vi "TDC_DAQV33_Paralled_muon.vi"(7 "address":string[](array[string])=["192.168.10.29"], 8 "error in (no error)":errorcluster, 9 "stop":bool, 10 "save data":bool=TRUE, 11 "SMA mode":bool) -> (0 "error out 3":errorcluster, 2 "csv path":path=path "G:/tdc/2017/data/test_20250707_095708.csv", 3 "rate":dbl=0.9919403977777173)   [LabVIEW 2017]
uses:
  gloabal.vi
  <vilib>/Utility/file.llb/Write Delimited Spreadsheet (DBL).vi
  <vilib>/Utility/file.llb/Write Delimited Spreadsheet (I64).vi
panel:
  in  "append csv 2":bool
  out "pmt trigger rate":u32[](array[numeric])=[0, 0, 1000, 0, 0, 0, 0, 0, 0, 0, 0, 0, 0, 0, 0, 0, 0, 0, 0, 0, 0, 0, 0, 0, 0, 0, 0, 0, 0, 0, 0, 0, 0, 0, 0, 0, 0, 0, 0, 0, 0, 0, 0, 0, 0, 0, 0, 0, 0, 0, 0, 0, 0, 0, 0, 0, 0, 0, 0, 0, 0, 0, 0, 0]
  out "event":u32[](array[numeric])=[0, 0, 0, 0, 1060, 1060, 0, 0, 0, 0, 0, 0, 0, 0, 0, 0, 0, 0, 0, 0, 0, 0, 0, 0, 0, 0, 0, 0, 0, 0, 0, 0, 0, 0, 0, 0, 0, 0, 0, 0, 0, 0, 0, 0, 0, 0, 0, 0, 0, 0, 0, 0, 0, 0, 0, 0, 0, 0, 0, 0, 0, 0, 0, 0, 0, 0, 0, 0, 0, 0, 0, 0, 0, 0, 0, 0, 0, 0, 0, 0, 0, 0, 0, 0, 0, 0, 0, 0, 0, 0, 0, 0, 0, 0, 0, 0, 0, 0, 0, 0, 0, 0, 0, 0, 0, 0, 0, 0, 0, 0, 0, 0, 0, 0, 0, 0, 0, 0, 0, 0, 0, 0, 0, 0, 0, 0, 0, 0]
  in  "calib_file":path=path "G:/tdc/2017/data/112_20250410_codeDensity.csv" caption="文件路径 （空时为对话框）"
  in  "use_calib_file":bool=TRUE
  out "second stamp":u64
  in  "coarse counter width":u16(ring) items=["29", "48"]
  out "name (unnamed)":string="Z\t"
  out "error out 5":errorcluster
  in  "timeout":dbl=30000.0
  out "DAC":dbl=8094.0
  out "Out":u8=3 format="%.0x"
  out "coarse":u64=407532724 format="%x"
  in  "gps":bool
  out "Year":string="2025"
  in  "factor":i32=128
  in  "displayCR":bool=TRUE
  in  "Counter Setting":dbl=100000.0 format="%#_13g"
  in  "replace dat":bool
  in  "append csv":bool=TRUE
  out "element":string
  out "fine":u64=646 format="%x"
  in  "UDP Config":bool=TRUE
  in  "data  path":path=path "G:/tdc/2017/data"
  out "cal 2":u64[](graph)
  in  "Thresholds (mV)":dbl[](array[numeric])=[580.0, 580.0, 580.0, 580.0, 600.0, 600.0, 600.0, 600.0, 580.0, 580.0, 600.0, 600.0, 600.0, 600.0, 600.0, 600.0, 580.0, 580.0, 600.0, 600.0, 600.0, 600.0, 600.0, 600.0, 580.0, 580.0, 600.0, 600.0, 600.0, 600.0, 600.0, 600.0, 600.0, 600.0, 600.0, 600.0, 600.0, 600.0, 600.0, 600.0, 600.0, 600.0, 600.0, 600.0, 600.0, 600.0, 600.0, 600.0, 600.0, 600.0, 600.0, 600.0, 600.0, 600.0, 600.0, 600.0, 600.0, 600.0, 600.0, 600.0, 600.0, 600.0, 600.0, 600.0]
  out "error out 2":errorcluster
  in  "display":bool=TRUE
  in  "Thresholds":dbl=-0.03
  in  "one key for threshold":bool=TRUE
  in  "RST":bool
  in  "通道数量":i32=128
  out "Cal Table":u32[](array[numeric])=[100002, 100002, 100002, 100002, 100002, 100002, 100002, 100002, 100002, 100002, 100002, 100002, 100002, 100002, 100002, 100002, 100002, 100002, 100002, 100002, 100002, 100002, 100002, 100002, 100002, 100002, 100002, 100002, 100002, 100002, 100002, 100002, 100002, 100002, 100002, 100002, 100002, 100002, 100002, 100002, 100002, 100002, 100002, 100002, 100002, 100002, 100002, 100002, 100002, 100002, 100002, 100002, 100002, 100002, 100002, 100002, 100002, 100002, 100002, 100002, 100002, 100002, 100002, 100002, 100002, 100002, 100002, 100002, 100002, 100002, 100002, 100002, 100002, 100002, 100002, 100002, 100002, 100002, 100002, 100002, 100002, 100002, 100002, 100002, 100002, 100002, 100002, 100002, 100002, 100002, 100002, 100002, 100002, 100002, 100002, 100002, 100002, 100002, 100002, 100002, 100002, 100002, 100002, 100002, 100002, 100002, 100002, 100002, 100002, 100002, 100002, 100002, 100002, 100002, 100002, 100002, 100002, 100002, 100002, 100002, 100002, 100002, 100002, 100002, 100002, 100002, 100002, 100002]
  in  "channel for cal":i32
  out "channel number":u64=5
  out "Calibration Counter":i32=536
  out "Event index":i32=97959
  out "cal":i64[](graph)=[0, 0, 0, 0, 0, 0, 0, 0, 0, 0, 0, 0, 0, 0, 0, 0, 0, 0, 0, 0, 0, 0, 0, 0, 0, 0, 0, 0, 0, 0, 0, 0, 0, 0, 0, 0, 0, 0, 0, 0, 0, 0, 0, 0, 0, 0, 0, 0, 0, 0, 0, 0, 0, 0, 0, 0, 0, 0, 0, 0, 0, 0, 0, 0, 0, 0, 0, 0, 0, 0, 0, 0, 0, 0, 0, 0, 0, 0, 0, 0, 0, 0, 0, 0, 0, 0, 0, 0, 0, 0, 0, 0, 0, 0, 0, 0, 0, 0, 0, 0, 0, 0, 0, 0, 0, 0, 0, 0, 0, 0, 0, 0, 0, 0, 0, 0, 0, 0, 0, 0, 0, 0, 0, 0, 0, 0, 0, 0, 0, 0, 0, 0, 0, 0, 0, 0, 0, 1, 76, 599, 343, 108, 71, 417, 154, 260, 138, 496, 255, 81, 42, 120, 215, 68, 109, 755, 65, 198, 68, 46, 289, 113, 477, 47, 391, 38, 57, 219, 61, 197, 92, 551, 105, 63, 72, 376, 118, 80, 104, 342, 66, 364, 53, 205, 180, 55, 61, 98, 566, 70, 259, 156, 66, 67, 62, 104, 344, 46, 318, 61, 43, 100, 186, 168, 212, 388, 97, 172, 75, 128, 55, 98, 77, 117, 184, 418, 122, 97, 132, 56, 45, 166, 426, 71, 70, 199, 69, 200, 161, 248, 119, 436, 79, 44, 50, 173, 567, 316, 65, 121, 253, 131, 217, 41, 55, 98, 38, 288, 113, 48, 254, 53, 28, 49, 132, 59, 311, 49, 49, 130, 54, 36, 46, 50, 158, 319, 298, 204, 87, 114, 100, 329, 92, 156, 15, 137, 321, 63, 192, 111, 45, 54, 43, 44, 598, 220, 210, 106, 235, 55, 49, 53, 377, 47, 32, 49, 50, 351, 179, 270, 239, 267, 89, 121, 85, 226, 33, 24, 25, 72, 480, 43, 48, 235, 221, 48, 66, 40, 422, 151, 110, 151, 177, 231, 74, 69, 108, 173, 239, 91, 371, 76, 80, 66, 459, 75, 238, 263, 522, 79, 63, 34, 80, 39, 64, 330, 323, 495, 47, 37, 33, 47, 399, 35, 32, 31, 100, 83, 44, 232, 44, 93, 144, 317, 125, 80, 64, 134, 85, 45, 156, 214, 71, 67, 406, 77, 45, 28, 35, 55, 136, 169, 99, 256, 128, 536, 80, 81, 92, 242, 165, 190, 64, 42, 72, 107, 301, 43, 55, 156, 281, 71, 245, 161, 73, 57, 387, 108, 146, 208, 61, 102, 266, 55, 224, 185, 56, 40, 83, 584, 66, 58, 46, 117, 163, 61, 303, 75, 85, 192, 150, 166, 72, 64, 161, 355, 147, 59, 195, 86, 71, 191, 55, 66, 353, 300, 73, 93, 202, 120, 66, 112, 284, 377, 166, 78, 145, 137, 190, 61, 48, 54, 277, 221, 458, 61, 69, 47, 366, 116, 215, 163, 64, 211, 129, 143, 119, 203, 426, 147, 228, 124, 116, 34, 101, 218, 59, 150, 117, 180, 58, 87, 231, 77, 150, 58, 106, 60, 226, 46, 46, 52, 371, 114, 275, 43, 41, 119, 67, 150, 60, 323, 211, 56, 94, 364, 108, 215, 52, 49, 150, 249, 240, 74, 119, 56, 298, 214, 132, 68, 81, 250, 114, 348, 87, 138, 63, 80, 423, 63, 67, 85, 224, 73, 245, 83, 38, 37, 181, 65, 312, 437, 138, 117, 42, 43, 105, 253, 82, 63, 86, 51, 175, 390, 48, 55, 377, 69, 117, 86, 498, 60, 54, 166, 214, 53, 100, 165, 77, 101, 205, 249, 342, 96, 522, 78, 45, 289, 230, 164, 363, 47, 56, 133, 76, 99, 133, 364, 83, 297, 109, 118, 78, 46, 35, 53, 215, 107, 62, 92, 81, 368, 47, 60, 168, 57, 110, 71, 58, 559, 141, 67, 113, 284, 287, 261, 134, 73, 53, 318, 104, 156, 632, 39, 27, 42, 433, 326, 279, 111, 229, 73, 91, 258, 88, 180, 213, 107, 329, 211, 54, 202, 126, 60, 149, 116, 154, 90, 68, 53, 73, 53, 199, 223, 118, 68, 152, 90, 197, 104, 49, 83, 340, 263, 86, 80, 100, 225, 475, 104, 160, 119, 248, 157, 81, 204, 157, 139, 99, 266, 82, 38, 71, 203, 458, 99, 186, 77, 115, 67, 353, 58, 37, 409, 84, 60, 85, 83, 96, 212, 161, 411, 374, 66, 44, 66, 84, 120, 196, 33, 35, 61, 205, 418, 169, 58, 95, 84, 34, 220, 84, 92, 239, 105, 273, 220, 55, 414, 81, 129, 130, 96, 165, 75, 393, 336, 170, 64, 84, 76, 386, 679, 76, 57, 161, 55, 76, 374, 268, 134, 206, 91, 61, 55, 395, 367, 166, 65, 35, 56, 224, 59, 92, 116, 197, 126, 121, 126, 63, 85, 138, 56, 11, 109, 5, 0, 1, 0, 0, 0, 0, 0, 0, 0, 0, 0, 0, 0, 0, 0, 0, 0, 0, 0, 0, 0, 0, 0, 0, 0, 0, 0, 0, 0, 0, 0, 0, 0, 0, 0, 0, 0, 0, 0, 0, 0, 0, 0, 0, 0, 0, 0, 0, 0, 0, 0, 0, 0, 0, 0, 0, 0, 0, 0, 0, 0, 0, 0, 0, 0, 0, 0, 0, 0, 0, 0, 0, 0, 0, 0, 0, 0, 0, 0, 0, 0, 0, 0, 0, 0, 0, 0, 0, 0, 0, 0, 0, 0, 0, 0, 0, 0, 0, 0, 0, 0, 0, 0, 0, 0, 0, 0, 0, 0, 0, 0, 0, 0, 0, 0, 0, 0, 0, 0, 0, 0, 0, 0, 0, 0, 0, 0, 0, 0, 0, 0, 0, 0, 0, 0, 0, 0, 0, 0, 0, 0, 0, 0, 0, 0, 0, 0, 0, 0, 0, 0, 0, 0, 0, 0, 0, 0, 0, 0, 0, 0, 0, 0, 0, 0, 0, 0, 0, 0, 0, 0, 0, 0, 0, 0, 0, 0, 0, 0, 0, 0, 0, 0, 0, 0, 0, 0, 0, 0, 0, 0, 0, 0, 0, 0, 0, 0, 0, 0, 0, 0, 0, 0, 0, 0, 0, 0, 0, 0, 0, 0, 0, 0, 0, 0, 0, 0, 0, 0, 0, 0, 0, 0, 0, 0, 0, 0, 0, 0, 0, 0, 0, 0, 0, 0, 0, 0, 0, 0, 0, 0, 0, 0, 0, 0, 0, 0, 0, 0, 0, 0, 0, 0, 0, 0, 0, 0, 0, 0, 0, 0, 0, 0, 0, 0, 0, 0, 0, 0, 0, 0, 0, 0, 0, 0, 0, 0, 0, 0, 0, 0, 0, 0, 0, 0, 0, 0, 0, 0, 0, 0, 0, 0, 0, 0, 0, 0, 0, 0, 0, 0, 0, 0, 0, 0, 0, 0, 0, 0, 0, 0, 0, 0, 0, 0, 0, 0, 0, 0, 0, 0, 0, 0, 0, 0, 0, 0, 0, 0, 0, 0, 0, 0, 0, 0, 0, 0, 0, 0, 0, 0, 0, 0, 0, 0, 0, 0, 0, 0, 0, 0, 0, 0, 0, 0, 0, 0, 0, 0, 0, 0, 0, 0, 0, 0, 0, 0, 0, 0, 0, 0, 0, 0, 0, 0, 0, 0, 0, 0, 0, 0, 0, 0, 0, 0, 0, 0, 0, 0, 0, 0, 0, 0, 0, 0, 0, 0, 0, 0, 0, 0, 0, 0, 0, 0, 0, 0, 0, 0, 0, 0, 0, 0, 0, 0, 0, 0, 0, 0, 0, 0, 0, 0, 0, 0, 0, 0, 0, 0, 0, 0, 0, 0, 0, 0, 0, 0, 0, 0, 0, 0, 0, 0, 0, 0, 0, 0, 0, 0, 0, 0, 0, 0, 0, 0, 0, 0, 0, 0, 0, 0, 0, 0, 0, 0, 0, 0, 0, 0, 0, 0, 0, 0, 0, 0, 0, 0, 0, 0, 0, 0, 0, 0, 0, 0, 0, 0, 0, 0, 0, 0, 0, 0, 0, 0, 0, 0, 0, 0, 0, 0, 0, 0, 0, 0, 0, 0, 0, 0, 0, 0, 0, 0, 0, 0, 0, 0, 0, 0, 0, 0, 0, 0, 0, 0, 0, 0, 0, 0, 0, 0, 0, 0, 0, 0, 0, 0, 0, 0, 0, 0, 0, 0, 0, 0, 0, 0, 0, 0, 0, 0, 0, 0, 0, 0, 0, 0, 0, 0, 0, 0, 0, 0, 0, 0, 0, 0, 0, 0, 0, 0, 0, 0, 0, 0, 0, 0, 0, 0, 0, 0, 0, 0, 0, 0, 0, 0, 0, 0, 0, 0, 0, 0, 0, 0, 0, 0, 0, 0, 0, 0, 0, 0, 0, 0, 0, 0, 0, 0, 0, 0, 0, 0, 0, 0, 0, 0, 0, 0, 0, 0, 0, 0, 0, 0, 0, 0, 0, 0, 0, 0, 0, 0, 0, 0, 0, 0, 0, 0, 0, 0, 0, 0, 0, 0, 0, 0, 0, 0, 0, 0, 0, 0, 0, 0, 0, 0, 0, 0, 0, 0, 0, 0, 0, 0, 0, 0, 0, 0, 0, 0, 0, 0, 0, 0, 0, 0, 0, 0, 0, 0, 0, 0, 0, 0, 0, 0, 0, 0, 0, 0, 0, 0, 0, 0, 0, 0, 0, 0, 0, 0, 0, 0, 0, 0, 0, 0, 0, 0, 0, 0, 0, 0, 0, 0, 0, 0, 0, 0, 0, 0, 0, 0, 0, 0, 0, 0, 0, 0, 0, 0, 0, 0, 0, 0, 0, 0, 0, 0, 0, 0, 0, 0, 0, 0, 0, 0, 0, 0, 0, 0, 0, 0, 0, 0, 0, 0, 0, 0, 0, 0, 0, 0, 0, 0, 0, 0, 0, 0, 0, 0, 0, 0, 0, 0, 0, 0, 0, 0, 0, 0, 0, 0, 0, 0, 0, 0, 0, 0, 0, 0, 0, 0, 0, 0, 0, 0, 0, 0, 0, 0, 0, 0, 0, 0, 0, 0, 0, 0, 0, 0, 0, 0, 0, 0, 0, 0, 0, 0, 0, 0, 0, 0, 0, 0, 0, 0, 0, 0, 0, 0, 0, 0, 0, 0, 0, 0, 0, 0, 0, 0, 0, 0, 0, 0, 0, 0, 0, 0, 0, 0, 0, 0, 0, 0, 0, 0, 0, 0, 0, 0, 0, 0, 0, 0, 0, 0, 0, 0, 0, 0, 0, 0, 0, 0, 0, 0, 0, 0, 0, 0, 0, 0, 0, 0, 0, 0, 0, 0, 0, 0, 0, 0, 0, 0, 0, 0, 0, 0, 0, 0, 0, 0, 0, 0, 0, 0, 0, 0, 0, 0, 0, 0, 0, 0, 0, 0, 0, 0, 0, 0, 0, 0, 0, 0, 0, 0, 0, 0, 0, 0, 0, 0, 0, 0, 0, 0, 0, 0, 0, 0, 0, 0, 0, 0, 0, 0, 0, 0, 0, 0, 0, 0, 0, 0, 0, 0, 0, 0, 0, 0, 0, 0, 0, 0, 0, 0, 0, 0, 0, 0, 0, 0, 0, 0, 0, 0, 0, 0, 0, 0, 0, 0, 0, 0, 0, 0, 0, 0, 0, 0, 0, 0, 0, 0, 0, 0, 0, 0, 0, 0, 0, 0, 0, 0, 0, 0, 0, 0, 0, 0, 0, 0, 0, 0, 0, 0, 0, 0, 0, 0, 0, 0, 0, 0, 0, 0, 0, 0, 0, 0, 0, 0, 0, 0, 0, 0, 0, 0, 0, 0, 0, 0, 0, 0, 0, 0, 0, 0, 0, 0, 0, 0, 0, 0, 0, 0, 0, 0, 0, 0, 0, 0, 0, 0, 0, 0, 0, 0, 0, 0, 0, 0, 0, 0, 0, 0, 0, 0, 0, 0, 0, 0, 0, 0, 0, 0, 0, 0, 0, 0, 0, 0, 0, 0, 0, 0, 0, 0, 0, 0, 0, 0, 0, 0, 0, 0, 0, 0, 0, 0, 0, 0, 0, 0, 0, 0, 0, 0, 0, 0, 0, 0, 0, 0, 0, 0, 0, 0, 0, 0, 0, 0, 0, 0, 0, 0, 0, 0, 0, 0, 0, 0, 0, 0, 0, 0, 0, 0, 0, 0, 0, 0, 0, 0, 0, 0, 0, 0, 0, 0, 0, 0, 0, 0, 0, 0, 0, 0, 0, 0, 0, 0, 0, 0, 0, 0, 0, 0, 0, 0, 0, 0, 0, 0, 0, 0, 0, 0, 0, 0, 0, 0, 0, 0, 0, 0, 0, 0, 0, 0, 0, 0, 0, 0, 0, 0, 0, 0, 0, 0, 0, 0, 0, 0, 0, 0, 0, 0, 0, 0, 0, 0, 0, 0, 0, 0, 0, 0, 0, 0, 0, 0, 0, 0, 0, 0, 0, 0, 0, 0, 0, 0, 0, 0, 0, 0, 0, 0, 0, 0, 0, 0, 0, 0, 0, 0, 0, 0, 0, 0, 0, 0]
  out "error out":errorcluster={"status"=TRUE, "code"=1, "source"="Close File in TDC_DAQV33_Paralled_muon.vi"}
  out "appended path":path=path "G:/tdc/2017/data/test_20250707_095708.dat"
  in  "filename":string="test"
  in  "Events":i32=110000 min=1
  in  "timeout (ms)":i32=10000
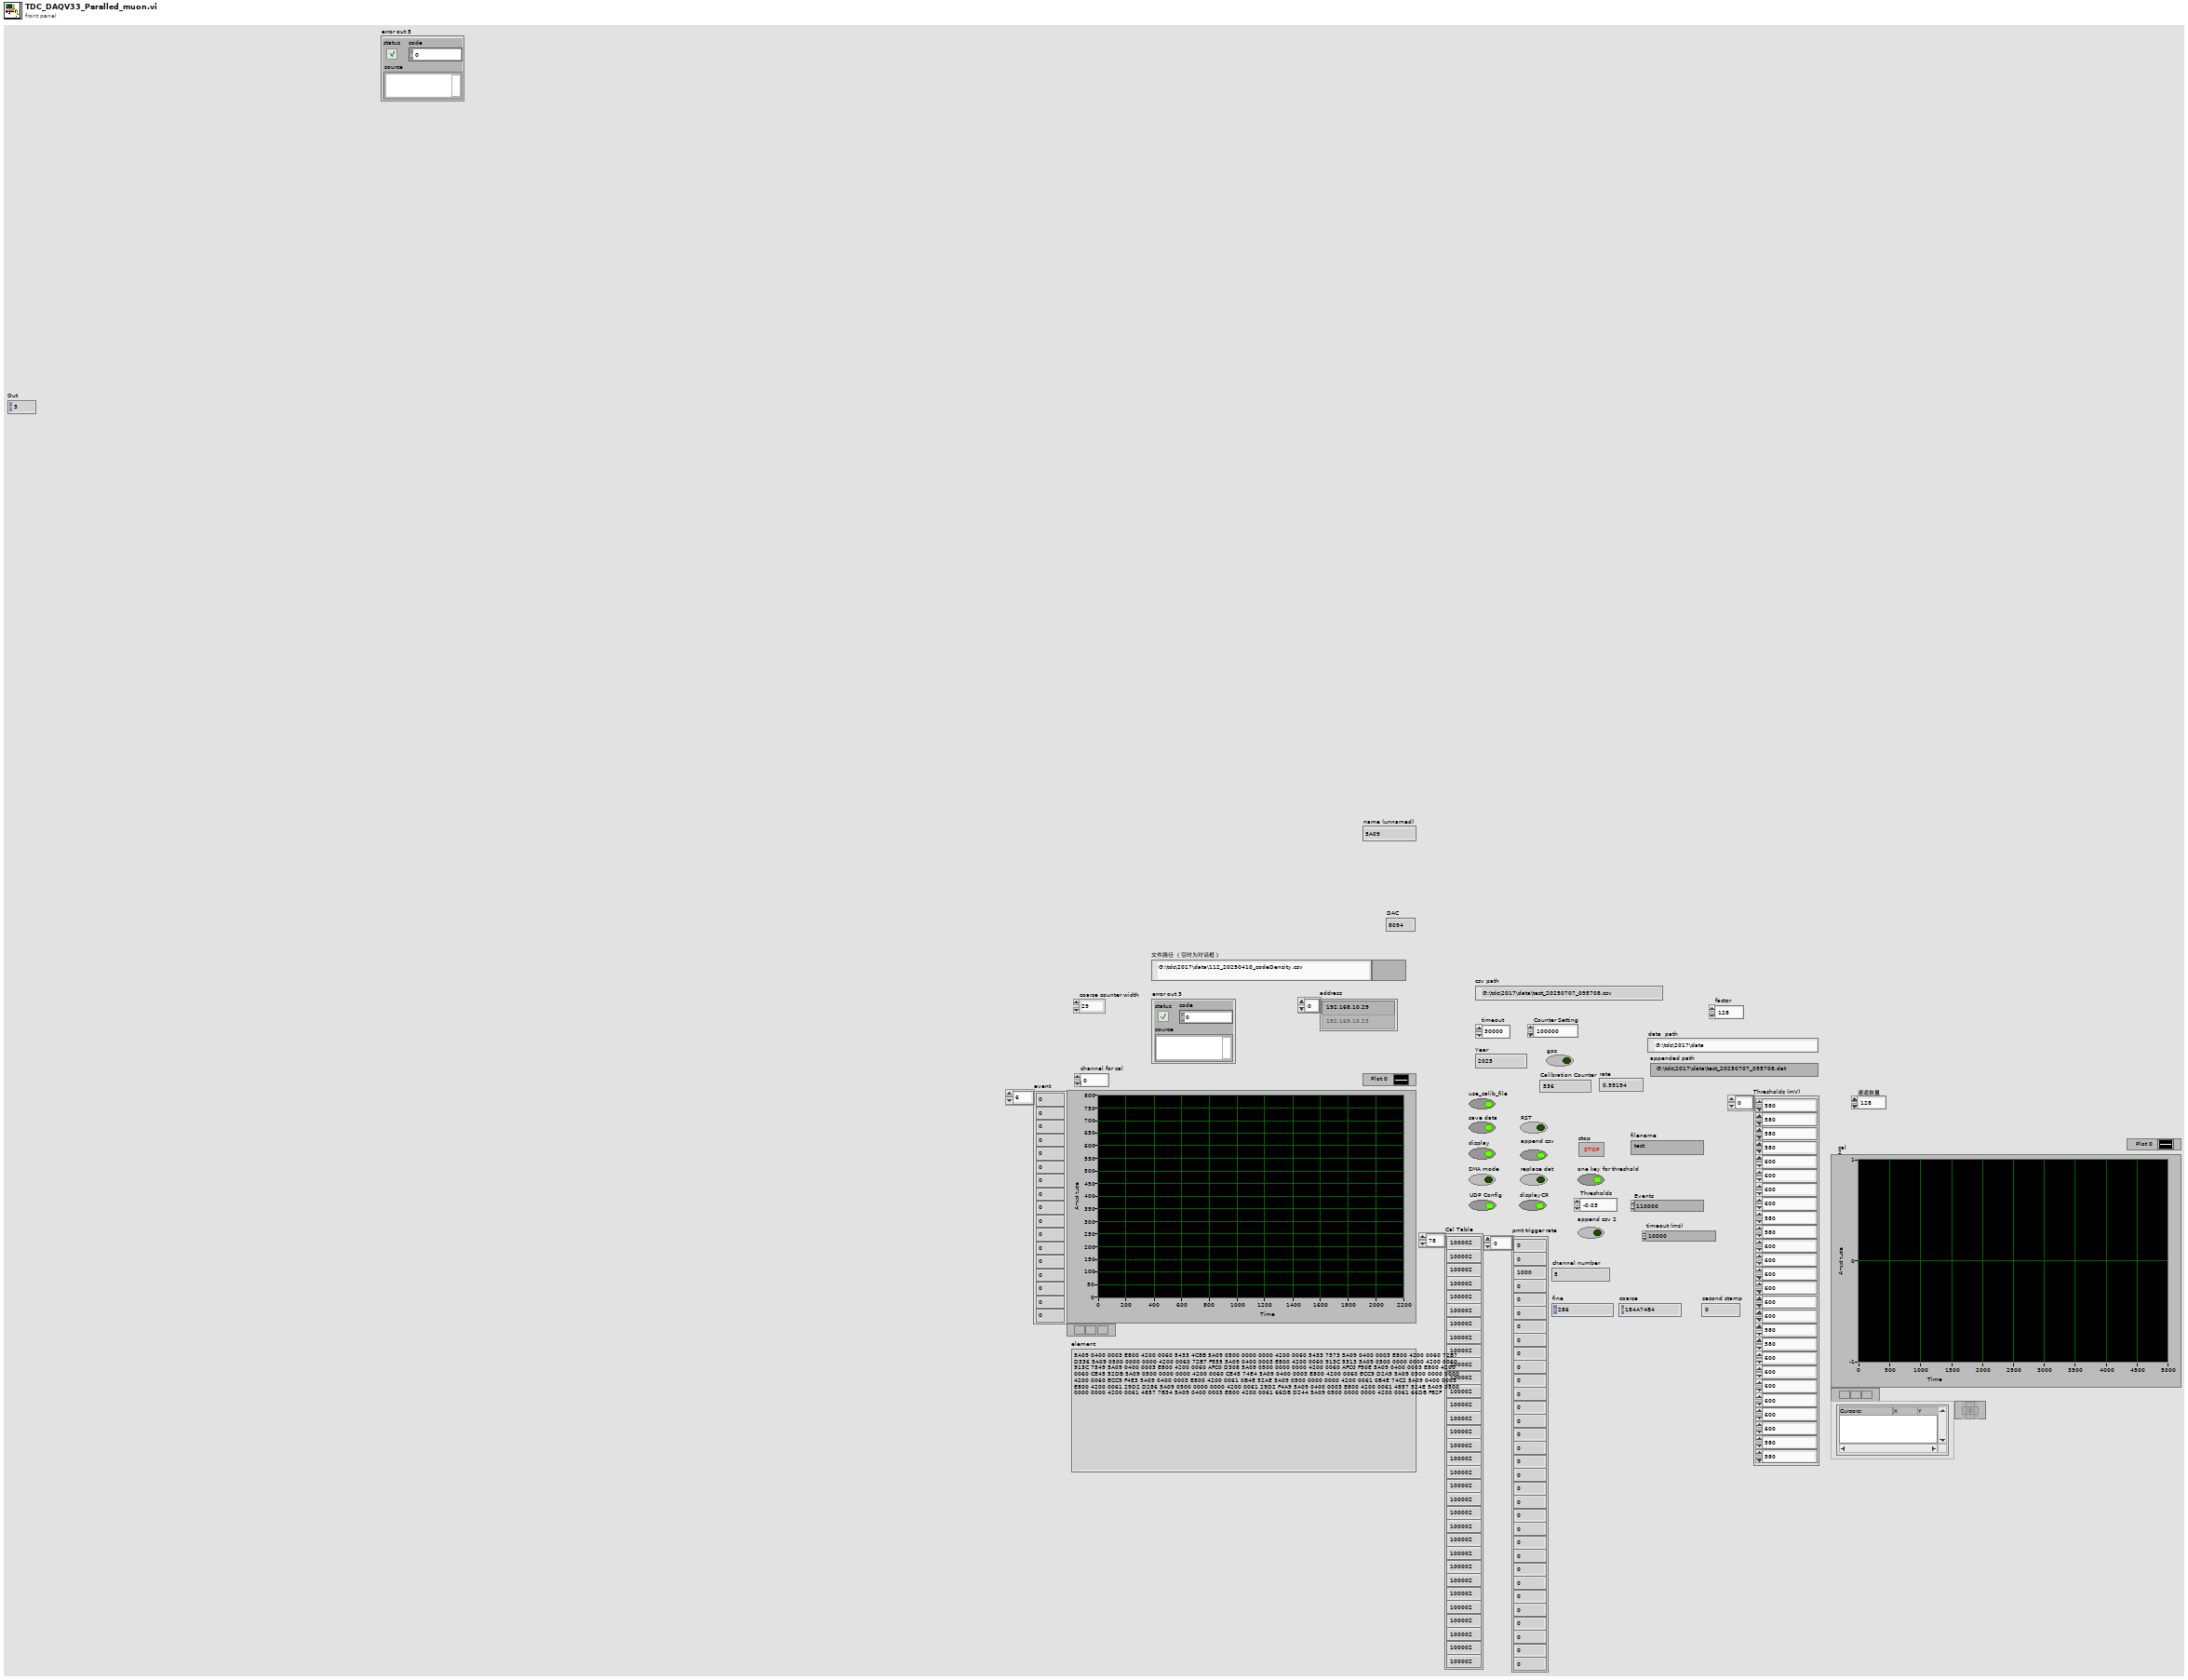
[diagram p1: front panel]
types:
  T1 = enum16{"open", "replace", "create", "open or create", "replace or create", "replace or create with confirmation"}
  T2 = enum16{"big-endian, network order", "native, host order", "little-endian"}
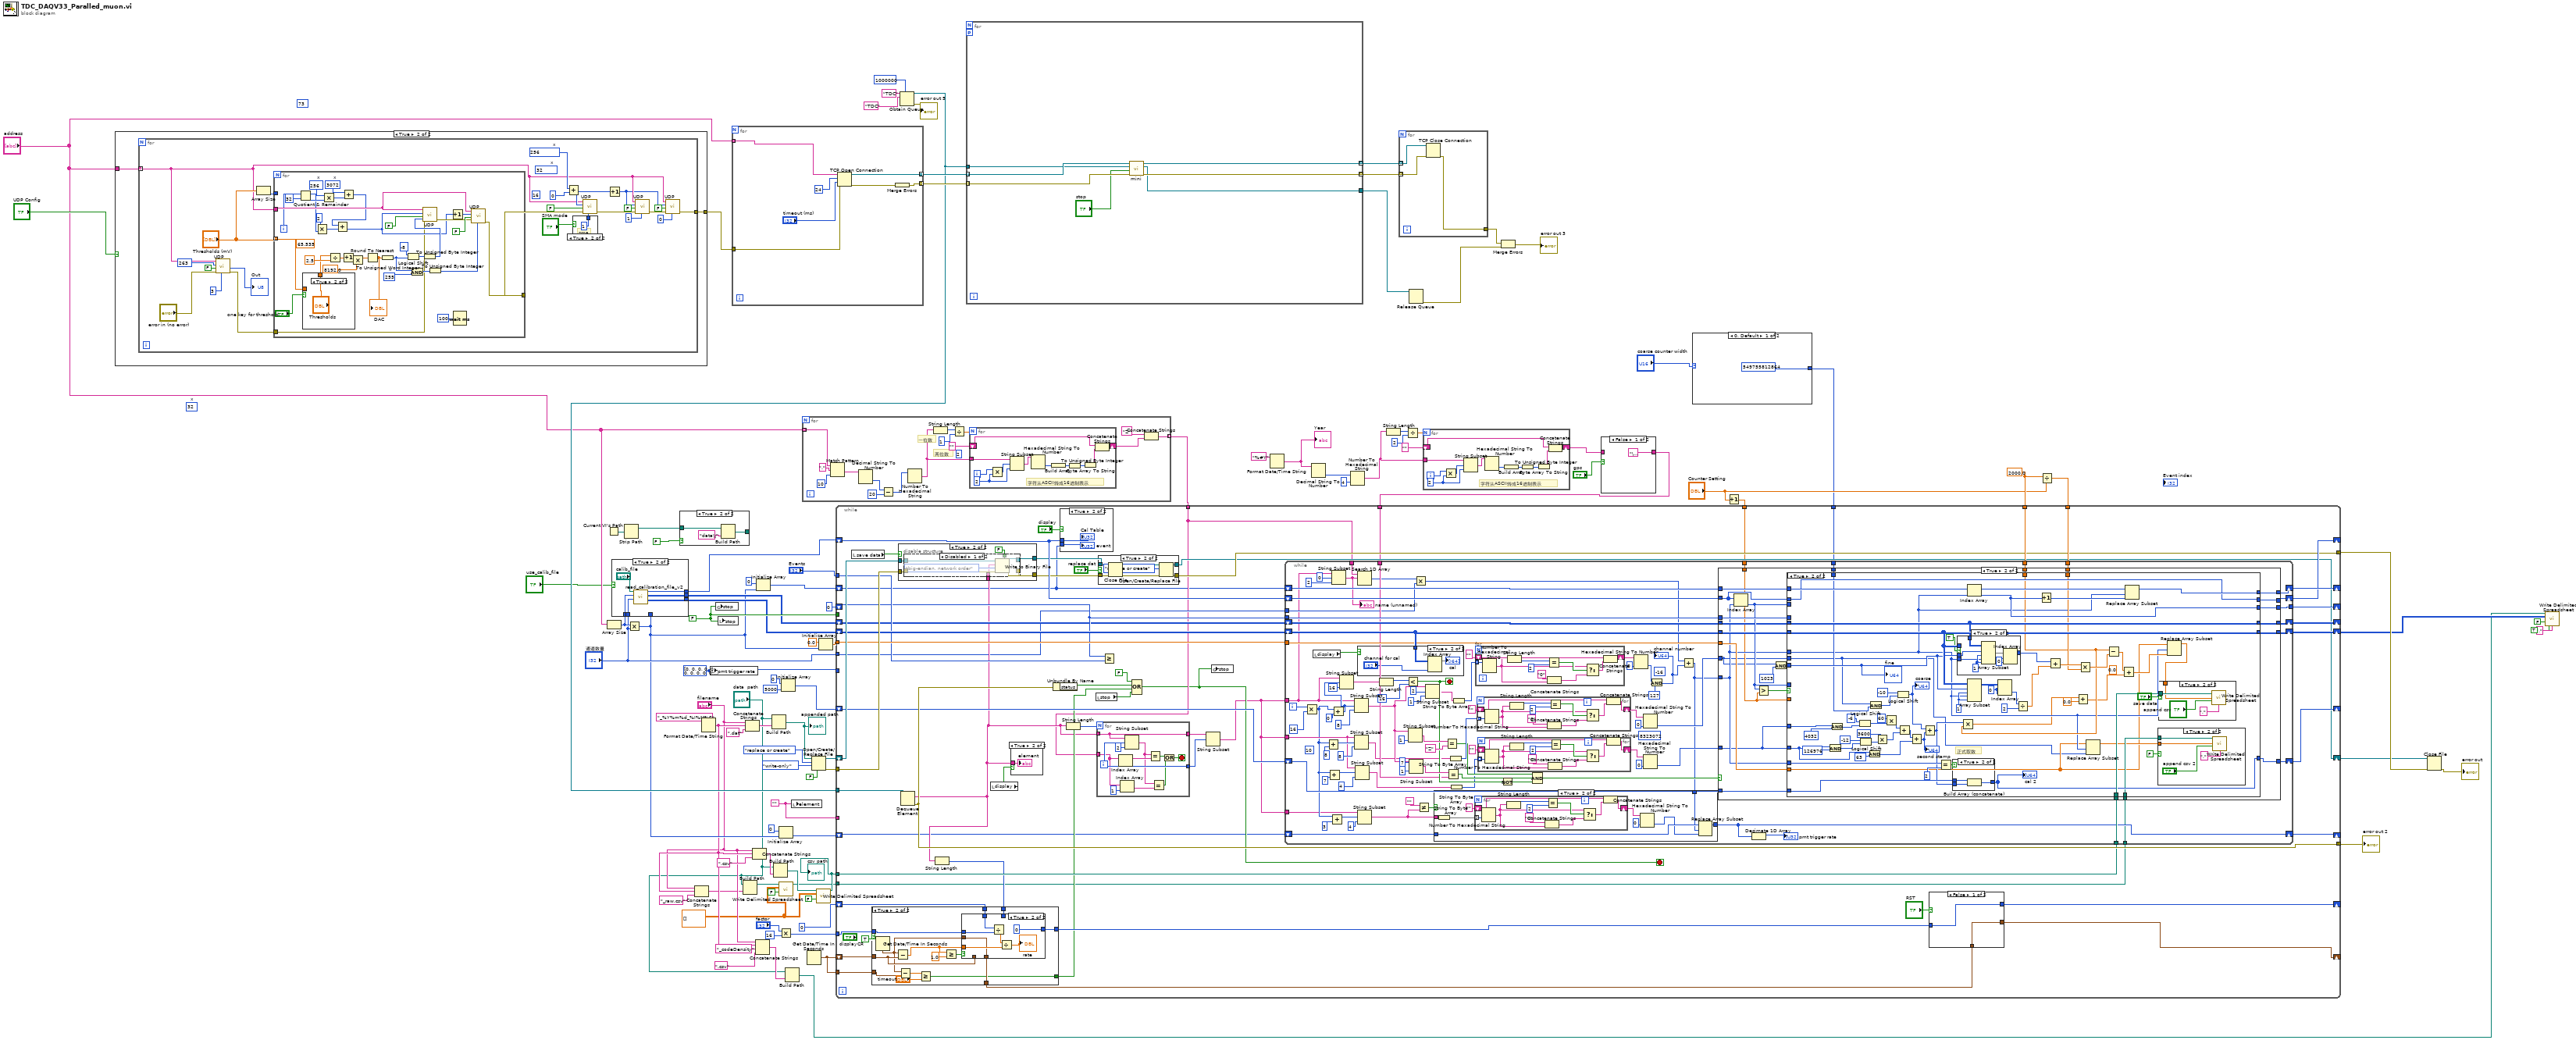
[diagram p0: block diagram]
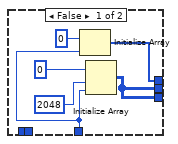
[diagram p2: hidden frame]
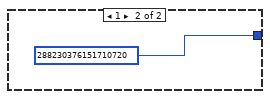
[diagram p3: hidden frame]
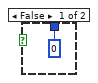
[diagram p6: hidden frame]
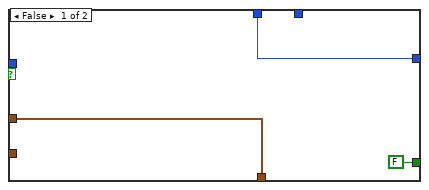
[diagram p13: hidden frame]
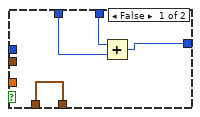
[diagram p14: hidden frame]
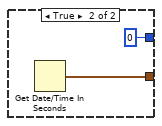
[diagram p16: hidden frame]
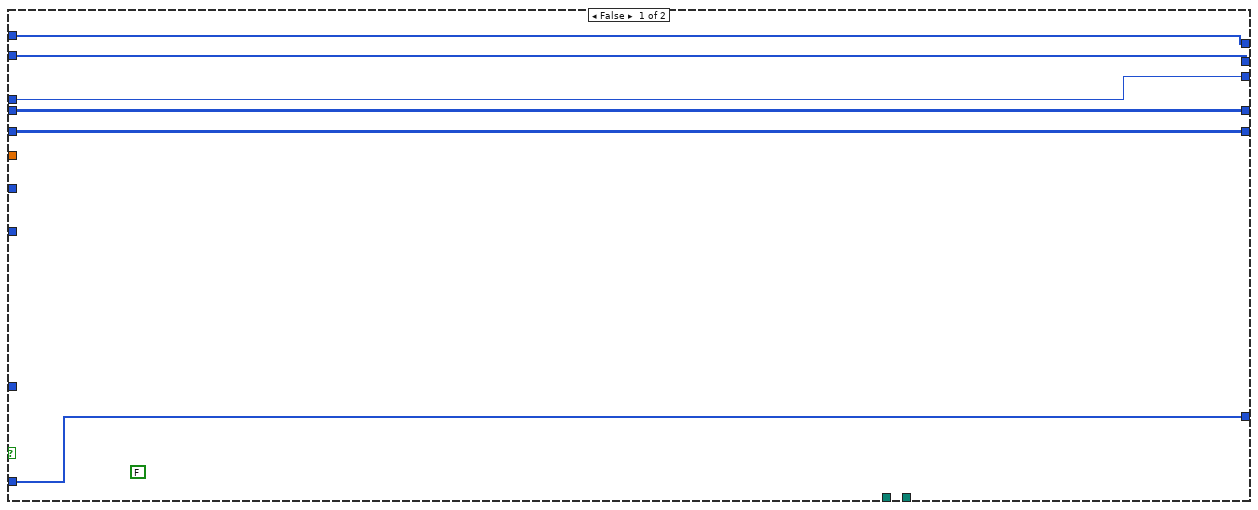
[diagram p19: hidden frame]
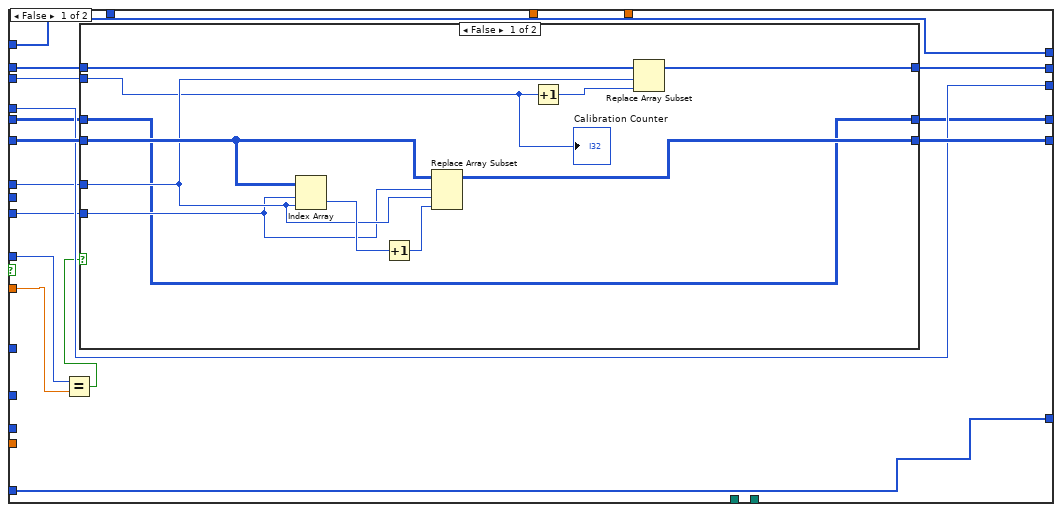
[diagram p20: hidden frame]
diagram:
  w10 = ""
  w11 = u32[] [0, 0, 0, 0, 0, 0, 0, 0, 0, 0, 0, 0, 0, 0, 0, 0, 0, 0, 0, 0, 0, 0, 0, 0, 0, 0, 0, 0, 0, 0, 0, 0, 0, 0, 0, 0, 0, 0, 0, 0, 0, 0, 0, 0, 0, 0, 0, 0, 0, 0, 0, 0, 0, 0, 0, 0, 0, 0, 0, 0, 0, 0, 0, 0] ("pmt trigger rate")
  (unwired) u32 73 ("Address")
  w62 = 2000.0 ("x")
  (unwired) u16 32  # x
  w24 = FALSE ("stop")
  w4 = dbl[][] [] ("2D data")
  n1 = case shown="True" "UDP Config" {
    tunnel: "address" -> [_ w100]
    tunnel: [_ w101] -> w29
    frame False {
    }
    frame True {
      n2 = for {
        tunnel: [w106] -> w101
        tunnel: w100 -> [w104] mode=indexing
        (unwired) u16 32  # x
        (unwired) u32 16 ("Address")
        w118 = u16 256  # x
        n3 = call "UDP.vi"("In"=u8 3, "error in (no error)"="error in (no error)", "Read (TRUE)"=FALSE, "Address"=u32 263, "IP address"=w104) -> ("error out"=w112:errorcluster, "Out"=→"Out":u8)  [unwired: 3 in, 1 out]
        n4 = Array Size(array="Thresholds (mV)") -> (size(s)=w121:i32)
        n5 = for {
          tunnel: w104 -> [w157]
          tunnel: "Thresholds (mV)" -> [w144] mode=indexing
          tunnel: [w147] -> w124
          tunnel: w121 -> [_]
          tunnel: w112 -> [w131]
          i -> [w139]
          (unwired) 65.535 ("y")
          w140 = u16 3072  # x
          w141 = u16 256  # x
          w153 = u16 255  # x
          n6 = Quotient & Remainder(x=w139, y=32) -> (x-y*floor(x/y)=w133:i32, floor(x/y)=w142:i32)
          n7 = case shown="True" "one key for threshold" {
            tunnel: [w163 "Thresholds"] -> w145
            tunnel: w144 -> [w163 _]
            frame False {
            }
            frame True {
            }
          }
          n8 = Multiply(x=2, y=w133) -> (x*y=w134:i32)
          n9 = Multiply(x=w141, y=w142) -> (x*y=w136:i32)
          n10 = Divide(x=w145, y=2.5) -> (x/y=w160:dbl)
          n11 = Increment(x=w160) -> (x+1=w130:dbl)
          n12 = Add(x=w140, y=w136) -> (x+y=w135:i32)
          n13 = Add(x=w135, y=w134) -> (x+y=w138:i32)
          n14 = Multiply(x=w130, y=8192.0) -> (x*y=w129:dbl)
          n15 = Round To Nearest(number=w129) -> (nearest integer value=w158:dbl)
          "DAC" <- w158
          n16 = To Unsigned Word Integer(number=w158) -> (unsigned 16bit integer=w149:u16)
          n17 = Logical Shift(y=i16 -8, x=w149) -> (x << y=w155:u16)
          n18 = And(x=w149, y=w153) -> (x .and. y?=w152:u16)
          n19 = To Unsigned Byte Integer(number=w155) -> (unsigned 8bit integer=w154:u8)
          n20 = call "UDP.vi"("In"=w154, "error in (no error)"=w131, "Read (TRUE)"=FALSE, "Address"=w138, "IP address"=w157) -> ("error out"=w148:errorcluster)  [unwired: 3 in, 2 out]
          n21 = To Unsigned Byte Integer(number=w152) -> (unsigned 8bit integer=w151:u8)
          n22 = Increment(x=w138) -> (x+1=w137:i32)
          n23 = Wait (ms)(milliseconds to wait=u32 100) -> ()  [unwired: 1 out]
          n24 = call "UDP.vi"("In"=w151, "error in (no error)"=w148, "Read (TRUE)"=FALSE, "Address"=w137, "IP address"=w157) -> ("error out"=w147:errorcluster)  [unwired: 3 in, 2 out]
        }
        n25 = Add(x=w118, y=u32 0 ("Address")) -> (x+y=w110:u32)
        n26 = case shown="True" "SMA mode" {
          tunnel: [u8 0 ("In") u8 1 ("In")] -> w123
          frame False {
          }
          frame True {
            # "sma"
          }
        }
        n27 = call "UDP.vi"("In"=w123, "error in (no error)"=w124, "Read (TRUE)"=FALSE, "Address"=w110, "IP address"=w104) -> ("error out"=w111:errorcluster)  [unwired: 3 in, 2 out]
        n28 = Increment(x=w110) -> (x+1=w103:u32)
        n29 = call "UDP.vi"("In"=u8 1, "error in (no error)"=w111, "Read (TRUE)"=FALSE, "Address"=w103, "IP address"=w104) -> ("error out"=w107:errorcluster)  [unwired: 3 in, 2 out]
        n30 = call "UDP.vi"("In"=u8 0, "error in (no error)"=w107, "Read (TRUE)"=FALSE, "Address"=w103, "IP address"=w104) -> ("error out"=w106:errorcluster)  [unwired: 3 in, 2 out]
      }
    }
  }
  n31 = Current VI's Path() -> (path=w94:path)
  n32 = Array Size(array="address") -> (size(s)=w16:i32)
  n33 = Strip Path(path=w94) -> (stripped path=w93:path)  [unwired: 1 out]
  n34 = Multiply(x=w16, y="通道数量") -> (x*y=w13:i32)
  n35 = case shown="True" "use_calib_file" {
    tunnel: w13 -> [w168 _]
    tunnel: [w165 w176] -> w19
    tunnel: [w165 w175] -> w18
    tunnel: [w166 w174] -> w17
    tunnel: w16 -> [_ w173]
    tunnel: "通道数量" -> [_ w172]
    frame False {
      n36 = Initialize Array(u32 0 ("element"), w168) -> (w166:u32[])
      n37 = Initialize Array(u32 0 ("element"), 2048 ("dimension size"), w168) -> (w165:u32[][])
    }
    frame True {
      n38 = call "read_calibration_file_v2.vi"("通道数量"=w172, "板子数量"=w173, "file path (dialog if empty)"="calib_file") -> ("code_density"=w176:i64[][], "accumulation"=w175:u32[][], "Cal Table"=w174:u32[])  [unwired: 5 in, 1 out]
    }
  }
  n39 = case shown="True" FALSE {
    tunnel: w93 -> [w177 w179]
    tunnel: [w177 w178] -> _
    frame False {
    }
    frame True {
      n40 = Build Path(base path=w179, name or relative path="data\\") -> (appended path=w178:path)
    }
  }
  n41 = Format Date/Time String(time format string (%c)="_%Y%m%d_%I%M%S") -> (date/time string=w8:string)  [unwired: 2 in]
  n42 = Concatenate Strings("filename", w8, "_raw.csv") -> (w6:string)
  n43 = local write "pmt trigger rate"(w11) -> ()
  n44 = global write "gloabal.vi" "stop"(w24) -> ()
  n45 = local write "stop"(w24) -> ()
  n46 = for {
    tunnel: "address" -> [w186] mode=indexing
    tunnel: [w185] -> w39 mode=indexing
    tunnel: [w183] -> w38 mode=indexing
    tunnel: w29 -> [w182]
    n47 = TCP Open Connection(address=w186, remote port or service name=u16 24 ("port"), timeout ms (60000)="timeout (ms)", error in (no error)=w182) -> (connection ID=w185:refnum<k5>, error out=w184:errorcluster)  [unwired: 1 in]
    n48 = Merge Errors(w184) -> (w183:errorcluster)
  }
  n49 = Build Path(base path="data  path", name or relative path=w6) -> (appended path=w1:path)
  n50 = Concatenate Strings("filename", w8, ".dat") -> (w92:string)
  n51 = Concatenate Strings("filename", w8, ".csv") -> (w82:string)
  n52 = Concatenate Strings("filename", w8, "_codeDensity" ("string"), ".csv") -> (w75:string)
  n53 = Initialize Array(u32 0 ("element"), w13) -> (w81:u32[])
  n54 = Build Path(base path="data  path", name or relative path=w92) -> (appended path=w91:path)
  "appended path" <- w91
  n55 = Build Path(base path="data  path", name or relative path=w82) -> (appended path=w80:path)
  n56 = Initialize Array(u32 0 ("element"), w13) -> (w12:u32[])
  n57 = call-poly <vilib>:"Write Delimited Spreadsheet.vi"("file path (dialog if empty)"=w1, "2D data"=w4, "append to file? (new file:F)"=FALSE) -> ("new file path (Not A Path if cancelled)"=w2:path)  [unwired: 11 in, 1 out]
  n58 = Multiply(x="factor", y=16) -> (x*y=w55:i32)
  n59 = Initialize Array(u32 0 ("element"), 5000 ("dimension size")) -> (w66:u32[])
  n60 = Build Path(base path="data  path", name or relative path=w75) -> (appended path=w72:path)
  n61 = local write "element"(w10) -> ()
  n62 = for {
    tunnel: [w189] -> w41 mode=indexing
    tunnel: "address" -> [w188] mode=indexing
    (unwired) 2 ("y")
    # "一位数"
    # "两位数"
    n63 = Match Pattern(string=w188, regular expression="." ("search string"), offset (0)=10) -> (after substring=w195:string)  [unwired: 3 out]
    n64 = Decimal String To Number(string=w195) -> (number=w192:i32)  [unwired: 2 in, 1 out]
    n65 = Subtract(x=w192, y=20) -> (x-y=w191:i32)
    n66 = Number To Hexadecimal String(2:w191) -> (0:w194:string)  [unwired: 1 in]
    n67 = String Length(string=w194) -> (length=w200:i32)
    n68 = Divide(x=w200, y=1) -> (x/y=w201:dbl)
    n69 = for {
      N: w201 -> [_]
      shift-right: [w213] -> w190
      shift-left: "" ("format string") -> [w212]
      tunnel: w194 -> [w203]
      i -> [w211]
      w205 = 2 ("y")
      # "字符从ASCII转成16进制表示"
      n70 = Multiply(x=w211, y=w205) -> (x*y=w204:i32)
      n71 = String Subset(string=w203, offset (0)=w204, length (rest)=w205) -> (substring=w206:string)
      n72 = Hexadecimal String To Number(string=w206) -> (number=w210:u32)  [unwired: 2 in, 1 out]
      n73 = Build Array(w210) -> (w209:u32[])
      n74 = To Unsigned Byte Integer(number=w209) -> (unsigned 8bit integer=w208:u8[])
      n75 = Byte Array To String(unsigned byte array=w208) -> (string=w207:string)
      n76 = Concatenate Strings(w212, w207) -> (w213:string)
    }
    n77 = Concatenate Strings("Z", w190) -> (w189:string)
  }
  n78 = Get Date/Time In Seconds() -> (seconds since 1Jan1904=w40:timestamp)
  n79 = Open/Create/Replace File(file path (use dialog)=w91, operation (0:open)=T1."replace or create", access (0:read/write)=enum16{"read/write", "read-only", "write-only"}."write-only", disable buffering (F)=FALSE) -> (refnum out=w96:refnum<file>, error out=w95:errorcluster)  [unwired: 2 in, 1 out]
  n80 = call-poly <vilib>:"Write Delimited Spreadsheet.vi"("file path (dialog if empty)"=w80, "2D data"=w4, "append to file? (new file:F)"=FALSE) -> ("new file path (Not A Path if cancelled)"=w23:path)  [unwired: 11 in, 1 out]
  "csv path" <- w23
  n81 = Initialize Array(0.0, w13) -> (w68:dbl[])
  n82 = Obtain Queue(max queue size (-1, unlimited)=1000000, name (unnamed)="TDC", element data type="TDC" ("name (unnamed)")) -> (queue out=w30:refnum<queue>, error out=→"error out 5":errorcluster)  [unwired: 2 in, 1 out]
  n83 = for {
    tunnel: w39 -> [w220] mode=indexing
    tunnel: w38 -> [w219] mode=indexing
    tunnel: [w218] -> w37 mode=indexing
    tunnel: [w217] -> w36 mode=indexing
    workers-P: _ -> [_]
    tunnel: w30 -> [w216]
    tunnel: [w215] -> w31
    n84 = call "mini.vi"("error in (no error)"=w219, "stop"="stop", "queue out 2"=w216, "connection ID 2"=w220) -> ("error out 3"=w217:errorcluster, "queue out"=w215:refnum<queue>, "connection ID"=w218:refnum<k5>)  [unwired: 5 in]
  }
  n85 = Format Date/Time String(time format string (%c)="%#Y") -> (date/time string=w52:string)  [unwired: 2 in]
  "Year" <- w52
  n86 = Decimal String To Number(string=w52) -> (number=w51:i32)  [unwired: 2 in, 1 out]
  n87 = Number To Hexadecimal String(1:i16 4 ("width (-)"), 2:w51) -> (0:w45:string)
  n88 = String Length(string=w45) -> (length=w47:i32)
  n89 = for {
    tunnel: w37 -> [w223] mode=indexing
    tunnel: w36 -> [w222] mode=indexing
    tunnel: [w221] -> w28
    n90 = TCP Close Connection(connection ID=w223, error in (no error)=w222) -> (error out=w221:errorcluster)  [unwired: 1 in, 1 out]
  }
  n91 = Divide(x=w47, y=2) -> (x/y=w48:dbl)
  n92 = Release Queue(queue=w31) -> (error out=w27:errorcluster)  [unwired: 2 in, 2 out]
  n93 = for {
    N: w48 -> [_]
    shift-right: [w234] -> w44
    shift-left: "" ("format string") -> [w233]
    tunnel: w45 -> [w224]
    i -> [w232]
    w226 = 2 ("y")
    # "字符从ASCII转成16进制表示"
    n94 = Multiply(x=w232, y=w226) -> (x*y=w225:i32)
    n95 = String Subset(string=w224, offset (0)=w225, length (rest)=w226) -> (substring=w227:string)
    n96 = Hexadecimal String To Number(string=w227) -> (number=w231:u32)  [unwired: 2 in, 1 out]
    n97 = Build Array(w231) -> (w230:u32[])
    n98 = To Unsigned Byte Integer(number=w230) -> (unsigned 8bit integer=w229:u8[])
    n99 = Byte Array To String(unsigned byte array=w229) -> (string=w228:string)
    n100 = Concatenate Strings(w233, w228) -> (w234:string)
  }
  n101 = Merge Errors(w28, w27) -> (→"error out 3":errorcluster)
  n102 = case shown="False" "gps" {
    tunnel: w44 -> [_ w236]
    tunnel: ["\u0000" ("format string") w236] -> w43
    frame False {
    }
    frame True {
    }
  }
  n103 = case shown="0, Default" "coarse counter width" {
    tunnel: [u64 549755812864 ("port") u64 288230376151710720 ("port")] -> w21
    frame 0, Default {
    }
    frame 1 {
    }
  }
  n104 = Increment(x="Counter Setting") -> (x+1=w58:dbl)
  n105 = Divide(x=w62, y="Counter Setting") -> (x/y=w61:dbl)
  n106 = while {
    tunnel: w95 -> [w296]
    tunnel: [w277] -> w69
    tunnel: [w266] -> w88
    shift-right: [w293] -> w73
    shift-left: w19 -> [w294]
    tunnel: "Events" -> [w291]
    shift-right: [w290] -> _
    shift-left: w81 -> [w243]
    shift-right: [w289] -> _
    shift-left: u32 0 ("element") -> [w288]
    shift-right: [w287] -> _
    shift-left: w17 -> [w279]
    shift-right: [w281] -> _
    shift-left: w18 -> [w286]
    tunnel: w23 -> [w273]
    shift-right: [w285] -> _
    shift-left: 0 -> [w260]
    shift-right: [w283] -> _
    shift-left: w40 -> [w282]
    tunnel: w24 -> [_]
    tunnel: w30 -> [w278]
    shift-right: [w274] -> _
    shift-left: w66 -> [w275]
    tunnel: w41 -> [w247]
    tunnel: w62 -> [w271]
    tunnel: w61 -> [w270]
    shift-right: [w265] -> w60
    shift-left: w96 -> [w295]
    tunnel: w58 -> [w264]
    tunnel: w55 -> [w257]
    tunnel: w43 -> [w255]
    tunnel: w40 -> [w254]
    tunnel: "通道数量" -> [w248]
    tunnel: w21 -> [w244]
    shift-right: [w240] -> _
    shift-left: w12 -> [w241]
    tunnel: w11 -> [_]
    tunnel: w10 -> [_]
    tunnel: w2 -> [w239]
    tunnel: w68 -> [w292]
    stop <- w246 stop-if-true
    n107 = local read "save data"() -> (w259:bool)
    n108 = Dequeue Element(queue=w278) -> (element=w250:string, error out=w277:errorcluster)  [unwired: 2 in, 2 out]
    n109 = case shown="True" w259 {
      tunnel: w296 -> [w309 w316]
      tunnel: w295 -> [w310 w315]
      tunnel: w250 -> [_ w313]
      tunnel: [w310 w312] -> w269
      tunnel: [w309 w311] -> w267
      frame False {
      }
      frame True {
        n110 = disable-structure shown="Disabled" {
          disable-tunnel: w316 -> [w323 _]
          disable-tunnel: w315 -> [w322 _]
          disable-tunnel: FALSE ("prepend array or string size? (T)") -> [w320 _]
          disable-tunnel: w313 -> [w319 _]
          disable-tunnel: [w318 _] -> w312
          disable-tunnel: [w317 _] -> w311
          frame Disabled {
            n111 = Write to Binary File(file (use dialog)=w322, data=w319, error in=w323, 5:w320, 9:T2."big-endian, network order" ("byte order (0:big-endian, network order)")) -> (refnum out=w318:refnum<file>, error out=w317:errorcluster)  [unwired: 1 in, 1 out]
          }
          frame Enabled {
          }
        }
      }
    }
    n112 = String Length(string=w250) -> (length=w261:i32)
    n113 = case shown="True" TRUE {
      tunnel: w282 -> [w335 w345]
      tunnel: [w335 w346] -> w263
      tunnel: w260 -> [w334 w344]
      tunnel: w261 -> [_ w343]
      tunnel: [w334 w342] -> w262
      tunnel: w257 -> [_ w341]
      tunnel: w254 -> [_ w339]
      tunnel: [FALSE w336] -> w253
      frame False {
      }
      frame True {
        n114 = Get Date/Time In Seconds() -> (seconds since 1Jan1904=w340:timestamp)
        n115 = Subtract(x=w340, y=w345) -> (x-y=w348:dbl)
        n116 = Subtract(x=w340, y=w339) -> (x-y=w338:dbl)
        n117 = Greater Or Equal?(x=w338, y="timeout") -> (x >= y?=w336:bool)
        n118 = Greater Or Equal?(x=w348, y=1.0) -> (x >= y?=w349:bool)
        n119 = case shown="True" w349 {
          tunnel: w348 -> [_ w360]
          tunnel: w340 -> [_ w358]
          tunnel: [w353 w358] -> w346
          tunnel: w345 -> [w353 _]
          tunnel: w344 -> [w352 w355]
          tunnel: w343 -> [w351 _]
          tunnel: [w350 0] -> w342
          tunnel: w341 -> [_ w354]
          frame False {
            n120 = Add(x=w351, y=w352) -> (x+y=w350:i32)
          }
          frame True {
            n121 = Divide(x=w355, y=w354) -> (x/y=w357:dbl)
            n122 = Divide(x=w357, y=w360) -> (x/y=→"rate":dbl)
          }
        }
      }
    }
    n123 = local read "display"() -> (w258:bool)
    n124 = case shown="True" w258 {
      tunnel: w250 -> [_ w308]
      frame False {
      }
      frame True {
        "element" <- w308
      }
    }
    n125 = Unbundle By Name(w277) -> ("status"=w276:bool)
    n126 = case shown="True" "display" {
      tunnel: w279 -> [_ w362]
      tunnel: w243 -> [_ w361]
      frame False {
      }
      frame True {
        "Cal Table" <- w362
        "event" <- w361
      }
    }
    n127 = String Length(string=w250) -> (length=w252:i32)
    n128 = local read "stop"() -> (w245:bool)
    n129 = for {
      N: w252 -> [_]
      tunnel: w250 -> [w305]
      tunnel: [w305] -> w251
      tunnel: [w304] -> w249
      tunnel: w247 -> [w302]
      i -> [w304]
      stop <- w298 stop-if-true
      n130 = Index Array(array=w302) -> (element=w303:string)  [unwired: 1 in]
      n131 = Index Array(array=w302, index=1) -> (element=w300:string)
      n132 = String Subset(string=w305, offset (0)=w304, length (rest)=2 ("length (rest)")) -> (substring=w299:string)
      n133 = Equal?(x=w299, y=w303) -> (x = y?=w306:bool)
      n134 = Equal?(x=w299, y=w300) -> (x = y?=w297:bool)
      n135 = Or(x=w306, y=w297) -> (x .or. y?=w298:bool)
    }
    n136 = case shown="True" "replace dat" {
      tunnel: w269 -> [w325 w331]
      tunnel: [w325 w330] -> w265
      tunnel: w267 -> [w324 w327]
      tunnel: [w324 w326] -> w266
      frame False {
      }
      frame True {
        n137 = Close File(refnum=w331, error in=w327) -> (path=w332:path, error out=w328:errorcluster)
        n138 = Open/Create/Replace File(file path (use dialog)=w332, error in=w328, operation (0:open)=T1."replace or create") -> (refnum out=w330:refnum<file>, error out=w326:errorcluster)  [unwired: 3 in, 1 out]
      }
    }
    n139 = Greater Or Equal?(x=w288, y=w291) -> ()  [unwired: 1 out]
    n140 = Compound Arithmetic op=OR(FALSE ("x"), w276, w253, w245) -> (w246:bool)
    n141 = String Subset(string=w251, offset (0)=w249) -> (substring=w242:string)  [unwired: 1 in]
    n142 = global write "gloabal.vi" "stop"(w246) -> ()
    n143 = while {
      tunnel: w242 -> [w384]
      shift-right: [w453] -> w293
      shift-left: w294 -> [w451]
      shift-right: [w447] -> w290
      shift-left: w243 -> [w446]
      tunnel: [w445] -> w289
      tunnel: w288 -> [w444]
      shift-right: [w442] -> w287
      shift-left: w279 -> [w443]
      tunnel: w273 -> [w440]
      shift-right: [w439] -> w281
      shift-left: w286 -> [w409]
      shift-right: [w436] -> w274
      shift-left: w275 -> [w437]
      tunnel: w242 -> [w403]
      tunnel: w271 -> [w416]
      tunnel: w270 -> [w415]
      tunnel: w264 -> [w408]
      tunnel: w255 -> [w398]
      tunnel: w248 -> [w386]
      tunnel: w247 -> [w385]
      tunnel: w244 -> [w381]
      tunnel: w242 -> [w371]
      shift-right: [w373] -> w240
      shift-left: w241 -> [w375]
      tunnel: w239 -> [w367]
      tunnel: w292 -> [w450]
      i -> [w454]
      stop <- w411 stop-if-true
      (unwired) 10 ("length (rest)")
      (unwired) u64 8323072 ("port")
      (unwired) i16 -16 ("y")
      n144 = Multiply(x=w454, y=16 ("length (rest)")) -> (x*y=w376:i32)
      n145 = local read "display"() -> (w438:bool)
      n146 = Add(x=w376, y=8 ("length (rest)")) -> (x+y=w428:i32)
      n147 = Add(x=w376, y=7 ("length (rest)")) -> (x+y=w405:i32)
      n148 = Add(x=w376, y=3 ("length (rest)")) -> (x+y=w378:i32)
      n149 = Add(x=w376, y=0 ("length (rest)")) -> (x+y=w414:i32)
      n150 = String Subset(string=w384, offset (0)=0, length (rest)=2 ("length (rest)")) -> (substring=w387:string)
      "name (unnamed)" <- w387
      n151 = String Subset(string=w384, offset (0)=w414, length (rest)=16 ("y")) -> (substring=w412:string)
      n152 = String Subset(string=w384, offset (0)=w414, length (rest)=8 ("length (rest)")) -> (substring=w396:string)
      n153 = String Subset(string=w403, offset (0)=w428, length (rest)=8 ("length (rest)")) -> (substring=w393:string)
      n154 = String Subset(string=w403, offset (0)=w405, length (rest)=4 ("length (rest)")) -> (substring=w392:string)
      n155 = Search 1D Array(1D array=w385, element=w387) -> (index of element=w388:i32)  [unwired: 1 in]
      n156 = case shown="True" w438 {
        tunnel: w451 -> [_ w500]
        frame False {
        }
        frame True {
          n157 = Index Array(array=w500, index (col)="channel for cal") -> (element=→"cal":i64[])  [unwired: 1 in]
        }
      }
      n158 = String Subset(string=w371, offset (0)=w378, length (rest)=4 ("length (rest)")) -> (substring=w369:string)
      n159 = String Length(string=w412) -> (length=w449:i32)
      n160 = Less?(x=w449, y=16) -> (x < y?=w411:bool)
      n161 = String Subset(string=w396, length (rest)=1 ("length (rest)")) -> (substring=w433:string)  [unwired: 1 in]
      n162 = String Subset(string=w396, offset (0)=7, length (rest)=1 ("length (rest)")) -> (substring=w417:string)
      n163 = Multiply(x=w388, y=w386) -> (x*y=w382:i32)
      n164 = Not Equal?(x="", y=w369) -> (x != y?=w370:bool)
      n165 = String Subset(string=w396, offset (0)=2, length (rest)=1 ("length (rest)")) -> (substring=w394:string)
      n166 = Equal?(x=w433, y="Z" ("format string")) -> (x = y?=w419:bool)
      n167 = Equal?(x=w417, y=w398) -> (x = y?=w418:bool)
      n168 = String To Byte Array(string=w393) -> (unsigned byte array=w425:u8[])
      n169 = String To Byte Array(string=w392) -> (unsigned byte array=w399:u8[])
      n170 = String To Byte Array(string=w394) -> (unsigned byte array=w456:u8[])
      n171 = for {
        shift-right: [w674] -> w422
        shift-left: "" ("format string") -> [w671]
        tunnel: w456 -> [w675] mode=indexing
        n172 = Number To Hexadecimal String(2:w675) -> (0:w667:string)  [unwired: 1 in]
        n173 = String Length(string=w667) -> (length=w673:i32)
        n174 = Equal?(x=w673, y=2) -> (x = y?=w670:bool)
        n175 = Concatenate Strings("0" ("format string"), w667) -> (w669:string)
        n176 = Select(t=w667, s=w670, f=w669) -> (s? t:f=w666:string)
        n177 = Concatenate Strings(w671, w666) -> (w674:string)
      }
      n178 = for {
        shift-right: [w496] -> w423
        shift-left: "" ("format string") -> [w488]
        tunnel: w425 -> [w497] mode=indexing
        n179 = Number To Hexadecimal String(2:w497) -> (0:w490:string)  [unwired: 1 in]
        n180 = String Length(string=w490) -> (length=w495:i32)
        n181 = Concatenate Strings("0" ("format string"), w490) -> (w492:string)
        n182 = Equal?(x=w495, y=2) -> (x = y?=w493:bool)
        n183 = Select(t=w490, s=w493, f=w492) -> (s? t:f=w489:string)
        n184 = Concatenate Strings(w488, w489) -> (w496:string)
      }
      n185 = for {
        shift-right: [w486] -> w402
        shift-left: "" ("format string") -> [w478]
        tunnel: w399 -> [w487] mode=indexing
        n186 = Number To Hexadecimal String(2:w487) -> (0:w480:string)  [unwired: 1 in]
        n187 = String Length(string=w480) -> (length=w485:i32)
        n188 = Concatenate Strings("0" ("format string"), w480) -> (w482:string)
        n189 = Equal?(x=w485, y=2) -> (x = y?=w483:bool)
        n190 = Select(t=w480, s=w483, f=w482) -> (s? t:f=w479:string)
        n191 = Concatenate Strings(w478, w479) -> (w486:string)
      }
      n192 = Not(x=w411) -> (.not. x?=w410:bool)
      n193 = Compound Arithmetic op=AND(w419, w418, w410) -> (w431:bool)
      n194 = Hexadecimal String To Number(string=w422, default (0uL)=u64 0 ("default (0 U32)")) -> (number=w452:u64)  [unwired: 1 in, 1 out]
      n195 = Hexadecimal String To Number(string=w423, default (0uL)=u64 0 ("default (0 U32)")) -> (number=w391:u64)  [unwired: 1 in, 1 out]
      n196 = Hexadecimal String To Number(string=w402, default (0uL)=u64 0 ("default (0 U32)")) -> (number=w380:u64)  [unwired: 1 in, 1 out]
      n197 = And(x=w452, y=u64 127 ("port")) -> (x .and. y?=w383:u64)
      "channel number" <- w383
      n198 = Add(x=w382, y=w383) -> (x+y=w374:u64)
      n199 = case shown="True" w370 {
        tunnel: w375 -> [w458 w464]
        tunnel: w374 -> [_ w462]
        tunnel: [w458 w461] -> w373
        tunnel: w369 -> [_ w460]
        frame False {
        }
        frame True {
          n200 = String To Byte Array(string=w460) -> (unsigned byte array=w465:u8[])
          n201 = for {
            shift-right: [w476] -> w459
            shift-left: "" ("format string") -> [w468]
            tunnel: w465 -> [w477] mode=indexing
            n202 = Number To Hexadecimal String(2:w477) -> (0:w470:string)  [unwired: 1 in]
            n203 = String Length(string=w470) -> (length=w475:i32)
            n204 = Concatenate Strings("0" ("format string"), w470) -> (w472:string)
            n205 = Equal?(x=w475, y=2) -> (x = y?=w473:bool)
            n206 = Select(t=w470, s=w473, f=w472) -> (s? t:f=w469:string)
            n207 = Concatenate Strings(w468, w469) -> (w476:string)
          }
          n208 = Hexadecimal String To Number(string=w459, default (0uL)=u64 0 ("default (0 U32)")) -> (number=w463:u64)  [unwired: 1 in, 1 out]
          n209 = Replace Array Subset(array=w464, new element=w463, index=w462) -> (w461:u32[])
        }
      }
      n210 = case shown="True" w431 {
        tunnel: w391 -> [_ w509]
        tunnel: w444 -> [w504 w524]
        tunnel: w451 -> [w506 w532]
        tunnel: [w506 w531] -> w453
        tunnel: w450 -> [_ w528]
        tunnel: w374 -> [_ w514]
        tunnel: w446 -> [w505 w527]
        tunnel: [w505 w526] -> w447
        tunnel: [w504 w525] -> w445
        tunnel: w443 -> [w503 w523]
        tunnel: [w503 w522] -> w442
        tunnel: w409 -> [w502 w520]
        tunnel: [w502 w519] -> w439
        tunnel: w440 -> [_ w518]
        tunnel: w437 -> [w501 w516]
        tunnel: [w501 w515] -> w436
        tunnel: w416 -> [_ w513]
        tunnel: w415 -> [_ w512]
        tunnel: w408 -> [_ w511]
        tunnel: w380 -> [_ w510]
        tunnel: w381 -> [_ w508]
        tunnel: w367 -> [_ w507]
        frame False {
          (unwired) FALSE
        }
        frame True {
          n211 = Index Array(array=w523, index=w514) -> (element=w521:u32)
          n212 = Greater?(x=w521, y=w511) -> (0:w517:bool)
          n213 = And(x=w509, y=u64 1023 ("port")) -> (x .and. y?=w529:u64)
          n214 = case shown="True" w517 {
            tunnel: w532 -> [w547 w628]
            tunnel: [w546 w628] -> w531
            tunnel: w529 -> [w539 w590]
            tunnel: w528 -> [_ w580]
            tunnel: w524 -> [w544 _]
            tunnel: w514 -> [w542 w582]
            tunnel: w527 -> [w545 w634]
            tunnel: [w545 w633] -> w526
            tunnel: [w544 w631] -> w525
            tunnel: w521 -> [w540 _]
            tunnel: w523 -> [w543 w630]
            tunnel: [w541 w630] -> w522
            tunnel: w521 -> [w537 _]
            tunnel: w511 -> [w534 _]
            tunnel: w520 -> [w536 w620]
            tunnel: [w535 w620] -> w519
            tunnel: w518 -> [_ w619]
            tunnel: w516 -> [w533 w616]
            tunnel: [w533 w615] -> w515
            tunnel: w514 -> [_ w612]
            tunnel: w513 -> [_ w610]
            tunnel: w512 -> [_ w611]
            tunnel: w510 -> [_ w605]
            tunnel: w510 -> [_ w594]
            tunnel: w509 -> [_ w579]
            tunnel: w508 -> [_ w588]
            tunnel: w507 -> [_ w583]
            frame False {
              n215 = Equal?(x=w537, y=w534) -> (x = y?=w538:bool)
              n216 = case shown="False" w538 {
                tunnel: w547 -> [w558 w564]
                tunnel: [w556 w564] -> w546
                tunnel: w543 -> [w554 w562]
                tunnel: w542 -> [w553 w559]
                tunnel: [w551 w561] -> w541
                tunnel: w540 -> [w550 w560]
                tunnel: w539 -> [w549 _]
                tunnel: w536 -> [w548 w566]
                tunnel: [w548 w565] -> w535
                frame False {
                  n217 = Index Array(array=w558, index (row)=w549, index (col)=w553) -> (element=w557:i64)
                  n218 = Increment(x=w557) -> (x+1=w555:i64)
                  n219 = Replace Array Subset(array=w558, new element=w555, index (row)=w549, index (col)=w553) -> (w556:i64[][])
                  n220 = Increment(x=w550) -> (x+1=w552:u32)
                  n221 = Replace Array Subset(array=w554, new element=w552, index=w553) -> (w551:u32[])
                  "Calibration Counter" <- w550
                }
                frame True {
                  n222 = for {
                    N: 2048 -> [_]
                    tunnel: w564 -> [w576]
                    tunnel: w559 -> [w569]
                    shift-right: [w571] -> w565
                    shift-left: w566 -> [w572]
                    i -> [w568]
                    n223 = Array Subset(array=w576, index (row)=0 ("索引"), length (row)=w568, index (col)=w569, length (col)=1 ("长度")) -> (w573:i64[][])
                    n224 = Add Array Elements(numeric array=w573) -> (sum=w570:i64)
                    n225 = Replace Array Subset(array=w572, new element=w570, index (row)=w568, index (col)=w569) -> (w571:u32[][])
                  }
                  n226 = Increment(x=w560) -> (x+1=w563:u32)
                  n227 = Replace Array Subset(array=w562, new element=w563, index=w559) -> (w561:u32[])
                }
              }
            }
            frame True {
              (unwired) 0.0 ("x")
              w625 = 0 ("索引 (行)")
              w627 = 1 ("长度")
              # "正式取数"
              n228 = And(x=w594, y=u64 126976 ("port")) -> (x .and. y?=w602:u64)
              n229 = And(x=w605, y=u64 4032 ("port")) -> (x .and. y?=w608:u64)
              n230 = Logical Shift(y=i16 -6, x=w608) -> (x << y=w591:u64)
              n231 = Logical Shift(y=i16 -12, x=w602) -> (x << y=w601:u64)
              n232 = And(x=w594, y=u64 63 ("port")) -> (x .and. y?=w584:u64)
              n233 = And(x=w579, y=w588) -> (x .and. y?=w589:u64)
              n234 = Multiply(x=u64 3600, y=w601) -> (x*y=w597:u64)
              n235 = Multiply(x=u64 60, y=w591) -> (x*y=w598:u64)
              n236 = Logical Shift(y=i16 -10, x=w589) -> (x << y=w586:u64)
              "coarse" <- w586
              n237 = Add(x=w598, y=w597) -> (x+y=w596:u64)
              n238 = Add(x=w596, y=w584) -> (x+y=w587:u64)
              "second stamp" <- w587
              n239 = Add(x=w586, y=w587) -> (x+y=w585:u64)
              n240 = Equal?(x=w612, y=u32 2) -> (x = y?=w614:bool)
              n241 = case shown="True" w614 {
                tunnel: w616 -> [w643 w646]
                tunnel: w585 -> [_ w645]
                tunnel: [w643 w644] -> w615
                frame False {
                }
                frame True {
                  n242 = Build Array (concatenate)(w646, w645) -> (w644:u64[])
                }
              }
              "cal 2" <- w615
              n243 = case shown="True" TRUE {
                tunnel: [w653 w661] -> w636
                tunnel: w628 -> [_ _]
                tunnel: w582 -> [w658 w659]
                tunnel: w590 -> [w656 w664]
                tunnel: w620 -> [w657 w665]
                frame False {
                  w652 = 0 ("index (row)")
                  w655 = 1 ("长度")
                  n244 = Decrement(x=w658) -> (x-1=w651:u64)
                  n245 = Array Subset(array=w657, index (row)=w656, length (row)=w655, index (col)=w651, length (col)=w655) -> (w654:u32[][])
                  n246 = Index Array(array=w654, index (row)=w652, index (col)=w652) -> (element=w653:u32)
                }
                frame True {
                  w660 = 0 ("index (row)")
                  w663 = 1 ("长度")
                  n247 = Array Subset(array=w665, index (row)=w664, length (row)=w663, index (col)=w659, length (col)=w663) -> (w662:u32[][])
                  n248 = Index Array(array=w662, index (row)=w660, index (col)=w660) -> (element=w661:u32)
                }
              }
              n249 = Multiply(x=w585, y=w610) -> (x*y=w578:dbl)
              n250 = Index Array(array=w634, index=w582) -> (element=w631:u32)
              n251 = Array Subset(array=w628, index (row)=w590, length (row)=w627, index (col)=w582, length (col)=w627) -> (w626:i64[][])
              n252 = Index Array(array=w626, index (row)=w625, index (col)=w625) -> (element=w624:i64)
              n253 = Divide(x=w624, y=u32 2) -> (x/y=w629:dbl)
              n254 = Increment(x=w631) -> (x+1=w632:u32)
              n255 = Add(x=w636, y=w629) -> (x+y=w635:dbl)
              n256 = Add(x=w578, y=0.0) -> (x+y=w593:dbl)
              n257 = Multiply(x=w635, y=w611) -> (x*y=w622:dbl)
              n258 = Replace Array Subset(array=w580, new element=w579, index=w582) -> (w581:dbl[])
              n259 = Subtract(x=w610, y=w622) -> (x-y=w609:dbl)
              n260 = Add(x=w609, y=w593) -> (x+y=w623:dbl)
              n261 = Replace Array Subset(array=w634, new element=w632, index=w582) -> (w633:u32[])
              n262 = case shown="True" FALSE {
                tunnel: w583 -> [_ w640]
                tunnel: w581 -> [_ w639]
                frame False {
                }
                frame True {
                  n263 = call-poly <vilib>:"Write Delimited Spreadsheet.vi"("file path (dialog if empty)"=w640, "1D data"=w639, "append to file? (new file:F)"="append csv 2", "delimiter (\\t)"="," ("delimiter (\\t)")) -> ()  [unwired: 10 in, 2 out]
                }
              }
              n264 = Replace Array Subset(array=w580, new element=w623, index=w582) -> (w618:dbl[])
              n265 = case shown="True" "save data" {
                tunnel: w619 -> [_ w650]
                tunnel: w618 -> [_ w648]
                frame False {
                }
                frame True {
                  n266 = call-poly <vilib>:"Write Delimited Spreadsheet.vi"("file path (dialog if empty)"=w650, "1D data"=w648, "append to file? (new file:F)"="append csv", "delimiter (\\t)"="," ("delimiter (\\t)")) -> ()  [unwired: 10 in, 2 out]
                }
              }
              "fine" <- w590
            }
          }
        }
      }
      n267 = Decimate 1D Array(w373) -> (→"pmt trigger rate":u32[])  [unwired: 1 out]
    }
    n268 = case shown="False" "RST" {
      tunnel: w262 -> [w364 _]
      tunnel: [w364 0] -> w285
      tunnel: [w363 w365] -> w283
      tunnel: w263 -> [w363 _]
      frame False {
      }
      frame True {
        n269 = Get Date/Time In Seconds() -> (seconds since 1Jan1904=w365:timestamp)
      }
    }
  }
  "error out 2" <- w69
  n270 = Close File(refnum=w60, error in=w88) -> (error out=→"error out":errorcluster)  [unwired: 1 out]
  n271 = call-poly <vilib>:"Write Delimited Spreadsheet.vi"("file path (dialog if empty)"=w72, "2D data"=w73, "append to file? (new file:F)"=FALSE, "transpose? (no:F)"=TRUE, "delimiter (\\t)"="," ("delimiter (\\t)")) -> ()  [unwired: 9 in, 2 out]
